vi "Begin.vi"(11 "Image Size":T1=enum."160x120") -> (0 "error out":errorcluster)   [LabVIEW 2012]
doc: "Called before other user functions, this VI is expected to open initial I/O refnums, load in file data, and do all program initialization. Notice that the <B>error out</B> terminal is simply used for data flow. Wiring it to other structures or subVIs ensures that this VI runs first."
uses:
  <vilib>/Rock Robotics/WPI/Camera/WPI_CameraImageSize.ctl
  <vilib>/Rock Robotics/WPI/DriverStation/WPI_DriverStationRobotMode2.ctl
  <vilib>/Rock Robotics/WPI/CAN/Jaguar/SubVIs/WPI_CANJaguar_BrakeCoastMode.ctl
  <vilib>/Rock Robotics/WPI/CAN/Jaguar/SubVIs/WPI_CANJaguar_SpeedReference.ctl
  <vilib>/Rock Robotics/WPI/CAN/Jaguar/SubVIs/WPI_CANJaguar_ControlMode.ctl
  <vilib>/Rock Robotics/WPI/Joystick/WPI_JoystickDeviceEnum.ctl
  <vilib>/Rock Robotics/SystemInterfaces/Typedef/FPGA_TypedefDigitalModule.ctl
  <vilib>/Rock Robotics/SystemInterfaces/DIO/FPGA_DIOChannel.ctl
  <vilib>/Rock Robotics/SystemInterfaces/DIO/FPGA_DIORelayChannel.ctl
  <vilib>/Rock Robotics/SystemInterfaces/Typedef/FPGA_TypedefSolenoidModule.ctl
  <vilib>/Rock Robotics/WPI/Solenoid/WPI_SolenoidChannel.ctl
  <vilib>/Rock Robotics/WPI/Solenoid/WPI_SolenoidValue.ctl
  Robot Global Data.vi
  <vilib>/Rock Robotics/WPI/MotorControl/WPI_MotorControlOpenCANJaguar.vi
  <vilib>/Rock Robotics/WPI/RobotDrive/WPI_RobotDriveOpen4MotorWithExistingMotors.vi
  <vilib>/Rock Robotics/WPI/Solenoid/WPI_SolenoidOpenSingle.vi
  <vilib>/Rock Robotics/WPI/Solenoid/WPI_SolenoidSetEnum.vi
  <vilib>/Rock Robotics/WPI/Compressor/WPI_CompressorGetSetRefNum.vi
  <vilib>/Rock Robotics/WPI/RobotDrive/WPI_RobotDriveOpen2MotorWithJaguar.vi
  <vilib>/Rock Robotics/SystemInterfaces/DIO/FPGA_DIOPWMChannel.ctl
  <vilib>/Rock Robotics/WPI/Camera/WPI_CameraWhite Balance Values.ctl
  <vilib>/Rock Robotics/WPI/Camera/WPI_CameraExposure Values.ctl
  <vilib>/Rock Robotics/WPI/Camera/WPI_CameraFrameRate.ctl
  <vilib>/Rock Robotics/WPI/SafetyOutput/WPI_SafetyOutputConfigMenu.ctl
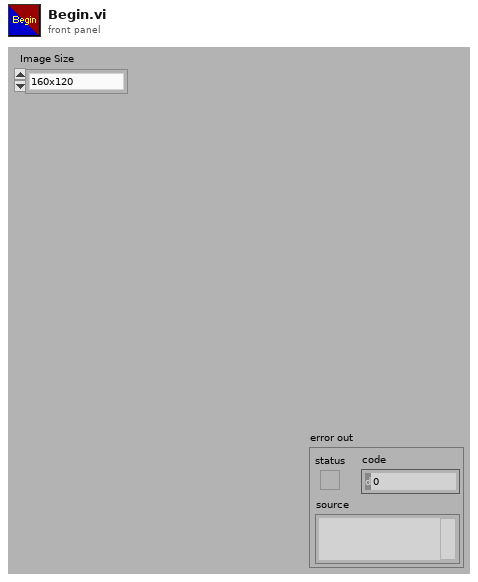
[diagram p1: front panel]
types:
  T1 = typedef "WPI_CameraImageSize.ctl" = enum16{"640x480", "320x240", "160x120"}
  T2 = typedef "WPI_SolenoidValue.ctl" = enum16{"Off", "On", "Forward", "Reverse"}
  T3 = typedef "WPI_SolenoidChannel.ctl" = enum8{"Solenoid 1", "Solenoid 2", "Solenoid 3", "Solenoid 4", "Solenoid 5", "Solenoid 6", "Solenoid 7", "Solenoid 8", "Invalid"}
  T4 = typedef "FPGA_TypedefSolenoidModule.ctl" = enum16{"Solenoid Module 1", "Solenoid Module 2"}
  T5 = typedef "FPGA_DIORelayChannel.ctl" = enum8{"Relay 1", "Relay 2", "Relay 3", "Relay 4", "Relay 5", "Relay 6", "Relay 7", "Relay 8", "Invalid"}
  T6 = typedef "FPGA_TypedefDigitalModule.ctl" = enum16{"Digital Module 1", "Digital Module 2"}
  T7 = typedef "FPGA_DIOChannel.ctl" = enum8{"DIO 1", "DIO 2", "DIO 3", "DIO 4", "DIO 5", "DIO 6", "DIO 7", "DIO 8", "DIO 9", "DIO 10", "DIO 11", "DIO 12", "DIO 13", "DIO 14", "Invalid"}
  T8 = typedef "WPI_JoystickDeviceEnum.ctl" = enum16{"USB 1", "USB 2", "USB 3", "USB 4", "Kinect 1", "Kinect 2"}
  T9 = typedef "WPI_CANJaguar_BrakeCoastMode.ctl" = enum8{"Jumper", "Brake", "Coast"}
  T10 = typedef "WPI_CANJaguar_SpeedReference.ctl" = u8
  T11 = typedef "WPI_CANJaguar_ControlMode.ctl" = enum8{"Percent VBus", "Current", "Speed", "Position", "Voltage"}
  T12 = typedef "WPI_DriverStationRobotMode2.ctl" = enum16{"Autonomous Disabled", "Autonomous Enabled", "Teleop Disabled", "Teleop Enabled", "Timeout", "Finish", "Test Disabled", "Test Enabled"}
  T13 = typedef "WPI_SafetyOutputConfigMenu.ctl" = enum16{"Enable", "Disable"}
  T14 = typedef "WPI_CameraFrameRate.ctl" = u32
  T15 = typedef "WPI_CameraExposure Values.ctl" = enum16{"Auto", "Flicker-free 50 Hz", "Flicker-free 60 Hz", "Hold current"}
  T16 = typedef "WPI_CameraWhite Balance Values.ctl" = enum16{"Auto", "Fixed indoor", "Fixed outdoor 1", "Fixed outdoor 2", "Fixed fluorescent 1", "Fixed fluorescent 2", "Hold current"}
  T17 = typedef "FPGA_DIOPWMChannel.ctl" = enum8{"PWM 1", "PWM 2", "PWM 3", "PWM 4", "PWM 5", "PWM 6", "PWM 7", "PWM 8", "PWM 9", "PWM 10", "Invalid"}
  T18 = typedef "WPI_CameraDevRef.ctl" = cluster{"Camera Address":string, "CameraStatus":errorcluster, "Acquire Image Notifier":refnum<notifier>}
  T19 = typedef "WPI_JoystickDevRef.ctl" = cluster{"Device":T8}
  T20 = typedef "WPI_RobotDriveDevRef.ctl" = cluster{"DevStatus":errorcluster, "Motors[]":T21[], "Square Inputs":bool, "Max Output":dbl, "Isochronous":bool}
  T21 = typedef "WPI_MotorControlDeviceRef.ctl" = cluster{"DeviceStatus":errorcluster, "Type":enum16{"PWM", "CAN"}, "PWM":cluster{"Digital Module":T6, "PWM Channel":T17, "DeadBand":T22}, "CAN":cluster{"Device Number":u8, "Control Mode":T11, "Semaphore":T23, "Max Vout":dbl}, "Invert":bool, "TransformRef":T24, "InvTransformRef":T24}
  T22 = typedef "WPI_PWMDeadband.ctl" = cluster{"Name":string, "maxPositivePwm":i32, "minPositivePwm":i32, "centerPwm":i32, "maxNegativePwm":i32, "minNegativePwm":i32, "angularRange":u16}
  T23 = typedef "Semaphore RefNum" = refnum<k1>
  T24 = typedef "WPI_PWMTransform_ConPane.ctl" = refnum<vi>
  T25 = typedef "WPI_SolenoidDevRef.ctl" = cluster{"DevStatus":errorcluster, "Solenoid Module":T4, "Forward Solenoid Channel":T3, "Reverse Solenoid Channel":T3}
  T26 = typedef "WPI_CompressorDevRef.ctl" = cluster{"DevStatus":errorcluster, "DigitalInputDevRef":T27, "RelayDevRef":T28}
  T27 = typedef "WPI_DigitalInputDevRef.ctl" = cluster{"DevStatus":errorcluster, "DIO Channel":T7, "Digital Module":T6}
  T28 = typedef "WPI_RelayDevRef.ctl" = cluster{"DevStatus":errorcluster, "Relay Channel":T5, "Digital Module":T6, "Relay Direction":T29}
  T29 = typedef "WPI_RelayDirection.ctl" = enum16{"Both directions", "Forward only", "Reverse only"}
  T30 = typedef "WPI_SerialPortRef.ctl" = cluster{"DevStatus":errorcluster, "Serial Port Name":refnum<visa-resource-name>}
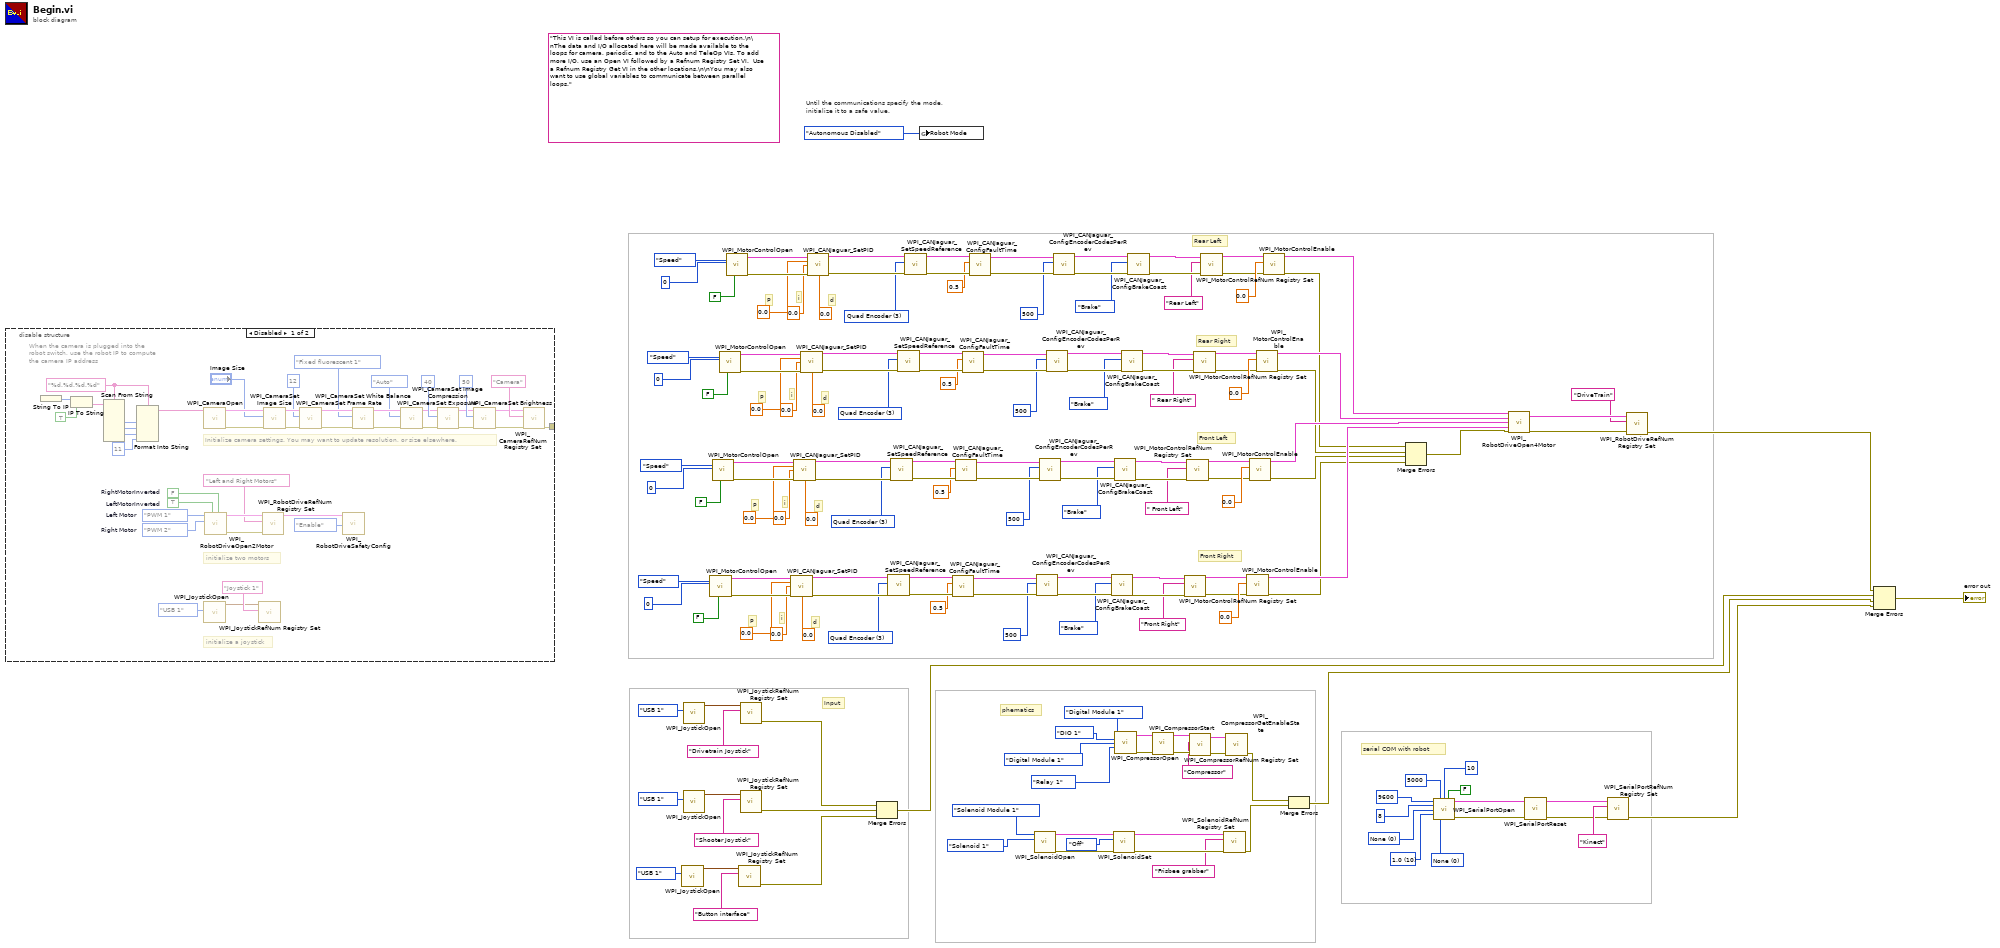
[diagram p0: block diagram]
diagram:
  w28 = u16 10 items=["1.0"=10, "1.5"=15, "2.0"=20] ("Stop Bits")
  w29 = u16 0 items=["None", "Odd", "Even", "Mark", "Space"] ("Parity")
  w32 = u16 0 items=["None", "XON/XOFF", "RTS/CTS", "XON/XOFF & RTS/CTS", "DTR/DSR", "XON/XOFF & DTR/DSR"] ("Flow Control")
  w76 = T10 3 items=["Encoder"=0, "Inv Encoder"=2, "Quad Encoder"=3, "None"=255] ("Speed Reference")
  w102 = T10 3 items=["Encoder"=0, "Inv Encoder"=2, "Quad Encoder"=3, "None"=255] ("Speed Reference")
  w128 = T10 3 items=["Encoder"=0, "Inv Encoder"=2, "Quad Encoder"=3, "None"=255] ("Speed Reference")
  w154 = T10 3 items=["Encoder"=0, "Inv Encoder"=2, "Quad Encoder"=3, "None"=255] ("Speed Reference")
  (unwired) "This VI is called before others so you can setup for execution.\n\nThe data and I/O allocated here will be made available to the loops for camera, periodic, and to the Auto and TeleOp VIs. To add more I/O, use an Open VI followed by a Refnum Registry Set VI.  Use a Refnum Registry Get VI in the other locations.\n\nYou may also want to use global variables to communicate between parallel loops."
  # "phematics"
  # "serial COM with robot"
  # "Input"
  # "Front Right"
  # "Front Left"
  # "Rear Right"
  # "Rear Left"
  # "d"
  # "i"
  # "P"
  # "d"
  # "i"
  # "P"
  # "d"
  # "i"
  # "P"
  # "d"
  # "i"
  # "P"
  # "Until the communications specify the mode,\ninitialize it to a safe value."
  n1 = disable-structure shown="Disabled" {
    disable-tunnel: [w169 _] -> _
    frame Disabled {
      w176 = "%d.%d.%d.%d" ("format string")
      w187 = FPGA_DIOPWMChannel."PWM 2"  # Right Motor
      w188 = FPGA_DIOPWMChannel."PWM 1"  # Left Motor
      w210 = TRUE  # LeftMotorInverted
      w211 = FALSE  # RightMotorInverted
      # "initialize a joystick"
      # "When the camera is plugged into the\nrobot switch, use the robot IP to compute\nthe camera IP address"
      # "initialize two motors"
      # "Initialize camera settings. You may want to update resolution, or size elsewhere."
      n2 = String To IP() -> (0:w183:u32)  [unwired: 1 in]
      n3 = IP To String(1:TRUE ("dot notation? (F)"), 2:w183) -> (0:w181:string)
      n4 = Scan From String(format string=w176, input string=w181) -> (output 1=w180:i32, output 2=w179:i32, output 3=w178:i32)  [unwired: 7 in, 3 out]
      n5 = Format Into String(format string=w176, w180, w179, w178, 11 ("Compression")) -> (resulting string=w173:string)  [unwired: 2 in, 1 out]
      n6 = call <vilib>:"WPI_CameraOpen.vi"("Camera Address"=w173) -> ("error out"=w197:errorcluster, "CameraDevRef"=w198:T18)  [unwired: 1 in, 8 out]
      n7 = call <vilib>:"WPI_JoystickOpen.vi"("JoystickDevice"=WPI_JoystickDeviceEnum."USB 1") -> ("JoystickDevRef"=w171:T19)  [unwired: 10 in]
      n8 = call-poly <vilib>:"WPI_RobotDriveOpen2Motor.vi"("Right Motor Inverted"=w211, "Left Motor Inverted"=w210, "Right Motor"=w187, "Left Motor"=w188) -> ("error out"=w206:errorcluster, "RobotDriveDevRef"=w208:T20)  [unwired: 1 in, 5 out]
      n9 = call <vilib>:"WPI_JoystickRefNum Registry Set.vi"("refnum name"="Joystick 1", "JoystickDevRef"=w171) -> ()  [unwired: 8 in, 2 out]
      n10 = call <vilib>:"WPI_RobotDriveRefNum Registry Set.vi"("error in (no error)"=w206, "refnum name"="Left and Right Motors", "RobotDriveDevRef"=w208) -> ("RobotDriveDevRef"=w175:T20)  [unwired: 8 out]
      n11 = call <vilib>:"WPI_CameraSet Image Size.vi"("error in (no error)"=w197, "Image Size"="Image Size", "CameraDevRef"=w198) -> ("error out"=w196:errorcluster, "CameraDevRef Out"=w199:T18)  [unwired: 7 out]
      n12 = call <vilib>:"WPI_CameraSet Frame Rate.vi"("error in (no error)"=w196, "Frame Rate (fps)"=T14 12, "CameraDevRef"=w199) -> ("error out"=w195:errorcluster, "CameraDevRef Out"=w201:T18)  [unwired: 7 out]
      n13 = call <vilib>:"WPI_RobotDriveSafetyConfig.vi"("mode"=WPI_SafetyOutputConfigMenu."Enable", "RobotDriveDevRef"=w175) -> ()  [unwired: 8 in, 2 out]
      n14 = call <vilib>:"WPI_CameraSet White Balance.vi"("error in (no error)"=w195, "White Balance"=WPI_CameraWhite_Balance_Values."Fixed fluorescent 1", "CameraDevRef"=w201) -> ("error out"=w194:errorcluster, "CameraDevRef Out"=w200:T18)  [unwired: 7 out]
      n15 = call <vilib>:"WPI_CameraSet Exposure.vi"("error in (no error)"=w194, "Exposure"=WPI_CameraExposure_Values."Auto", "CameraDevRef"=w200) -> ("error out"=w193:errorcluster, "CameraDevRef Out"=w203:T18)  [unwired: 7 out]
      n16 = call <vilib>:"WPI_CameraSet Image Compression.vi"("error in (no error)"=w193, "Compression"=40, "CameraDevRef"=w203) -> ("error out"=w192:errorcluster, "CameraDevRef Out"=w202:T18)  [unwired: 7 out]
      n17 = call <vilib>:"WPI_CameraSet Brightness.vi"("error in (no error)"=w192, "Brightness"=50, "CameraDevRef"=w202) -> ("error out"=w190:errorcluster, "CameraDevRef Out"=w191:T18)  [unwired: 7 out]
      n18 = call <vilib>:"WPI_CameraRefNum Registry Set.vi"("error in (no error)"=w190, "refnum name"="Camera", "CameraDevRef"=w191) -> ("error out"=w169:errorcluster)  [unwired: 8 out]
    }
    frame Enabled {
    }
  }
  n19 = call <vilib>:"WPI_JoystickOpen.vi"("JoystickDevice"=WPI_JoystickDeviceEnum."USB 1") -> ("JoystickDevRef"=w45:T19)  [unwired: 10 in]
  n20 = call <vilib>:"WPI_JoystickOpen.vi"("JoystickDevice"=WPI_JoystickDeviceEnum."USB 1") -> ("JoystickDevRef"=w51:T19)  [unwired: 10 in]
  n21 = call <vilib>:"WPI_JoystickOpen.vi"("JoystickDevice"=WPI_JoystickDeviceEnum."USB 1") -> ("JoystickDevRef"=w48:T19)  [unwired: 10 in]
  n22 = call-poly <vilib>:"WPI_MotorControlOpen.vi"("Invert"=FALSE, "Device Number"=u8 0, "Control Mode"=WPI_CANJaguar_ControlMode."Speed") -> ("error out"=w83:errorcluster, "MotorControlDeviceRef"=w82:T21)  [unwired: 7 in]
  n23 = call-poly <vilib>:"WPI_MotorControlOpen.vi"("Invert"=FALSE, "Device Number"=u8 0, "Control Mode"=WPI_CANJaguar_ControlMode."Speed") -> ("error out"=w109:errorcluster, "MotorControlDeviceRef"=w108:T21)  [unwired: 7 in]
  n24 = call-poly <vilib>:"WPI_MotorControlOpen.vi"("Invert"=FALSE, "Device Number"=u8 0, "Control Mode"=WPI_CANJaguar_ControlMode."Speed") -> ("error out"=w135:errorcluster, "MotorControlDeviceRef"=w134:T21)  [unwired: 7 in]
  n25 = call-poly <vilib>:"WPI_MotorControlOpen.vi"("Invert"=FALSE, "Device Number"=u8 0, "Control Mode"=WPI_CANJaguar_ControlMode."Speed") -> ("error out"=w161:errorcluster, "MotorControlDeviceRef"=w160:T21)  [unwired: 7 in]
  n26 = call <vilib>:"WPI_JoystickRefNum Registry Set.vi"("refnum name"="Button interface", "JoystickDevRef"=w45) -> ("error out"=w40:errorcluster)  [unwired: 8 in, 1 out]
  n27 = call <vilib>:"WPI_JoystickRefNum Registry Set.vi"("refnum name"="Drivetrain Joystick", "JoystickDevRef"=w51) -> ("error out"=w42:errorcluster)  [unwired: 8 in, 1 out]
  n28 = call <vilib>:"WPI_JoystickRefNum Registry Set.vi"("refnum name"="Shooter Joystick", "JoystickDevRef"=w48) -> ("error out"=w41:errorcluster)  [unwired: 8 in, 1 out]
  n29 = call <vilib>:"WPI_CANJaguar_SetPID.vi"("CAN Jaguar Ref"=w82, "P"=0.0, "I"=0.0, "D"=0.0, "error in (no error)"=w83) -> ("CAN Jaguar Ref Out"=w89:T21, "error out"=w88:errorcluster)  [unwired: 9 in]
  n30 = call <vilib>:"WPI_CANJaguar_SetPID.vi"("CAN Jaguar Ref"=w108, "P"=0.0, "I"=0.0, "D"=0.0, "error in (no error)"=w109) -> ("CAN Jaguar Ref Out"=w115:T21, "error out"=w114:errorcluster)  [unwired: 9 in]
  n31 = call <vilib>:"WPI_CANJaguar_SetPID.vi"("CAN Jaguar Ref"=w134, "P"=0.0, "I"=0.0, "D"=0.0, "error in (no error)"=w135) -> ("CAN Jaguar Ref Out"=w141:T21, "error out"=w140:errorcluster)  [unwired: 9 in]
  n32 = call <vilib>:"WPI_CANJaguar_SetPID.vi"("CAN Jaguar Ref"=w160, "P"=0.0, "I"=0.0, "D"=0.0, "error in (no error)"=w161) -> ("CAN Jaguar Ref Out"=w167:T21, "error out"=w166:errorcluster)  [unwired: 9 in]
  n33 = Merge Errors(w42, w41, w40) -> (w3:errorcluster)
  n34 = call <vilib>:"WPI_CANJaguar_SetSpeedReference.vi"("error in (no error)"=w88, "Speed Reference"=w76, "CAN Jaguar Ref"=w89) -> ("error out"=w87:errorcluster, "CAN Jaguar Ref Out"=w86:T21)  [unwired: 7 in]
  n35 = call <vilib>:"WPI_CANJaguar_SetSpeedReference.vi"("error in (no error)"=w114, "Speed Reference"=w102, "CAN Jaguar Ref"=w115) -> ("error out"=w113:errorcluster, "CAN Jaguar Ref Out"=w112:T21)  [unwired: 7 in]
  n36 = call <vilib>:"WPI_CANJaguar_SetSpeedReference.vi"("error in (no error)"=w140, "Speed Reference"=w128, "CAN Jaguar Ref"=w141) -> ("error out"=w139:errorcluster, "CAN Jaguar Ref Out"=w138:T21)  [unwired: 7 in]
  n37 = call <vilib>:"WPI_CANJaguar_SetSpeedReference.vi"("error in (no error)"=w166, "Speed Reference"=w154, "CAN Jaguar Ref"=w167) -> ("error out"=w165:errorcluster, "CAN Jaguar Ref Out"=w164:T21)  [unwired: 7 in]
  n38 = global write "Robot Global Data.vi" "Robot Mode"(WPI_DriverStationRobotMode2."Autonomous Disabled" ("Robot Mode")) -> ()
  n39 = call <vilib>:"WPI_CANJaguar_ConfigFaultTime.vi"("error in (no error)"=w87, "Fault Time (s)"=0.5, "CAN Jaguar Ref"=w86) -> ("error out"=w84:errorcluster, "CAN Jaguar Ref Out"=w85:T21)  [unwired: 7 in]
  n40 = call <vilib>:"WPI_CANJaguar_ConfigFaultTime.vi"("error in (no error)"=w113, "Fault Time (s)"=0.5, "CAN Jaguar Ref"=w112) -> ("error out"=w110:errorcluster, "CAN Jaguar Ref Out"=w111:T21)  [unwired: 7 in]
  n41 = call <vilib>:"WPI_CANJaguar_ConfigFaultTime.vi"("error in (no error)"=w139, "Fault Time (s)"=0.5, "CAN Jaguar Ref"=w138) -> ("error out"=w136:errorcluster, "CAN Jaguar Ref Out"=w137:T21)  [unwired: 7 in]
  n42 = call <vilib>:"WPI_CANJaguar_ConfigFaultTime.vi"("error in (no error)"=w165, "Fault Time (s)"=0.5, "CAN Jaguar Ref"=w164) -> ("error out"=w162:errorcluster, "CAN Jaguar Ref Out"=w163:T21)  [unwired: 7 in]
  n43 = call-poly <vilib>:"WPI_SolenoidOpen.vi"("Solenoid Channel"=WPI_SolenoidChannel."Solenoid 1", "Solenoid Module (Module 1)"=FPGA_TypedefSolenoidModule."Solenoid Module 1") -> ("error out"=w11:errorcluster, "SolenoidDevRef"=w13:T25)  [unwired: 8 in]
  n44 = call <vilib>:"WPI_CANJaguar_ConfigEncoderCodesPerRev.vi"("error in (no error)"=w84, "Encoder Codes Per Rev"=u16 500, "CAN Jaguar Ref"=w85) -> ("error out"=w73:errorcluster, "CAN Jaguar Ref Out"=w72:T21)  [unwired: 7 in]
  n45 = call <vilib>:"WPI_CANJaguar_ConfigEncoderCodesPerRev.vi"("error in (no error)"=w110, "Encoder Codes Per Rev"=u16 500, "CAN Jaguar Ref"=w111) -> ("error out"=w99:errorcluster, "CAN Jaguar Ref Out"=w98:T21)  [unwired: 7 in]
  n46 = call <vilib>:"WPI_CANJaguar_ConfigEncoderCodesPerRev.vi"("error in (no error)"=w136, "Encoder Codes Per Rev"=u16 500, "CAN Jaguar Ref"=w137) -> ("error out"=w125:errorcluster, "CAN Jaguar Ref Out"=w124:T21)  [unwired: 7 in]
  n47 = call <vilib>:"WPI_CANJaguar_ConfigEncoderCodesPerRev.vi"("error in (no error)"=w162, "Encoder Codes Per Rev"=u16 500, "CAN Jaguar Ref"=w163) -> ("error out"=w151:errorcluster, "CAN Jaguar Ref Out"=w150:T21)  [unwired: 7 in]
  n48 = call <vilib>:"WPI_CANJaguar_ConfigBrakeCoast.vi"("error in (no error)"=w73, "Brake / Coast Mode"=WPI_CANJaguar_BrakeCoastMode."Brake", "CAN Jaguar Ref"=w72) -> ("error out"=w69:errorcluster, "CAN Jaguar Ref Out"=w70:T21)  [unwired: 7 in]
  n49 = call-poly <vilib>:"WPI_SolenoidSet.vi"("error in (no error)"=w11, "Value"=WPI_SolenoidValue."Off", "SolenoidDevRef"=w13) -> ("error out"=w10:errorcluster, "SolenoidDevRef"=w9:T25)  [unwired: 7 in]
  n50 = call <vilib>:"WPI_CANJaguar_ConfigBrakeCoast.vi"("error in (no error)"=w99, "Brake / Coast Mode"=WPI_CANJaguar_BrakeCoastMode."Brake", "CAN Jaguar Ref"=w98) -> ("error out"=w95:errorcluster, "CAN Jaguar Ref Out"=w96:T21)  [unwired: 7 in]
  n51 = call <vilib>:"WPI_CompressorOpen.vi"("Pressure Switch Digital Module (Module 1)"=FPGA_TypedefDigitalModule."Digital Module 1", "Pressure Switch DIO Channel"=FPGA_DIOChannel."DIO 1", "Relay Digital Module (Module 1)"=FPGA_TypedefDigitalModule."Digital Module 1", "Relay Channel"=FPGA_DIORelayChannel."Relay 1") -> ("CompressorDevRef"=w22:T26, "error out"=w21:errorcluster)  [unwired: 10 in]
  n52 = call <vilib>:"WPI_CANJaguar_ConfigBrakeCoast.vi"("error in (no error)"=w125, "Brake / Coast Mode"=WPI_CANJaguar_BrakeCoastMode."Brake", "CAN Jaguar Ref"=w124) -> ("error out"=w121:errorcluster, "CAN Jaguar Ref Out"=w122:T21)  [unwired: 7 in]
  n53 = call <vilib>:"WPI_CANJaguar_ConfigBrakeCoast.vi"("error in (no error)"=w151, "Brake / Coast Mode"=WPI_CANJaguar_BrakeCoastMode."Brake", "CAN Jaguar Ref"=w150) -> ("error out"=w147:errorcluster, "CAN Jaguar Ref Out"=w148:T21)  [unwired: 7 in]
  n54 = call <vilib>:"WPI_CompressorStart.vi"("error in (no error)"=w21, "CompressorDevRef"=w22) -> ("error out"=w26:errorcluster, "CompressorDevRef"=w25:T26)  [unwired: 8 in]
  n55 = call <vilib>:"WPI_MotorControlRefNum Registry Set.vi"("error in (no error)"=w69, "refnum name"="Front Right", "MotorControlDevRef"=w70) -> ("error out"=w64:errorcluster, "MotorControlDevRef"=w66:T21)  [unwired: 7 in]
  n56 = call <vilib>:"WPI_MotorControlRefNum Registry Set.vi"("error in (no error)"=w95, "refnum name"=" Front Left", "MotorControlDevRef"=w96) -> ("error out"=w90:errorcluster, "MotorControlDevRef"=w92:T21)  [unwired: 7 in]
  n57 = call <vilib>:"WPI_CompressorRefNum Registry Set.vi"("error in (no error)"=w26, "refnum name"="Compressor", "CompressorDevRef"=w25) -> ("error out"=w24:errorcluster, "CompressorDevRef"=w23:T26)  [unwired: 7 in]
  n58 = call <vilib>:"WPI_MotorControlRefNum Registry Set.vi"("error in (no error)"=w121, "refnum name"=" Rear Right", "MotorControlDevRef"=w122) -> ("error out"=w116:errorcluster, "MotorControlDevRef"=w118:T21)  [unwired: 7 in]
  n59 = call <vilib>:"WPI_MotorControlRefNum Registry Set.vi"("error in (no error)"=w147, "refnum name"="Rear Left", "MotorControlDevRef"=w148) -> ("error out"=w142:errorcluster, "MotorControlDevRef"=w144:T21)  [unwired: 7 in]
  n60 = call <vilib>:"WPI_SolenoidRefNum Registry Set.vi"("error in (no error)"=w10, "refnum name"="Frisbee grabber", "SolenoidDevRef"=w9) -> ("error out"=w6:errorcluster)  [unwired: 7 in, 1 out]
  n61 = call <vilib>:"WPI_CompressorGetEnableState.vi"("error in (no error)"=w24, "CompressorDevRef"=w23) -> ("error out"=w7:errorcluster)  [unwired: 6 in, 3 out]
  n62 = call <vilib>:"WPI_MotorControlEnable.vi"("error in (no error)"=w64, "Encoder Initial Position"=0.0, "CAN Jaguar Ref"=w66) -> ("error out"=w57:errorcluster, "CAN Jaguar Ref Out"=w60:T21)  [unwired: 7 in]
  n63 = call <vilib>:"WPI_MotorControlEnable.vi"("error in (no error)"=w90, "Encoder Initial Position"=0.0, "CAN Jaguar Ref"=w92) -> ("error out"=w56:errorcluster, "CAN Jaguar Ref Out"=w61:T21)  [unwired: 7 in]
  n64 = call <vilib>:"WPI_MotorControlEnable.vi"("error in (no error)"=w116, "Encoder Initial Position"=0.0, "CAN Jaguar Ref"=w118) -> ("error out"=w58:errorcluster, "CAN Jaguar Ref Out"=w62:T21)  [unwired: 7 in]
  n65 = call <vilib>:"WPI_MotorControlEnable.vi"("error in (no error)"=w142, "Encoder Initial Position"=0.0, "CAN Jaguar Ref"=w144) -> ("error out"=w59:errorcluster, "CAN Jaguar Ref Out"=w63:T21)  [unwired: 7 in]
  n66 = Merge Errors(w7, w6) -> (w2:errorcluster)
  n67 = Merge Errors(w59, w58, w56, w57) -> (w55:errorcluster)
  n68 = call <vilib>:"WPI_SerialPortOpen.vi"("Baud Rate"=u32 9600, "Timeout Value (ms)"=u32 5000, "Termination Char (0xA = '\\n' = LF)"=u8 10 ("Termination Char (0xA = '\\n' = LF)"), "Enable Termination Char? (T)"=FALSE, "Data Bits"=u16 8, "Parity"=w29, "Stop Bits"=w28, "Flow Control"=w32) -> ("SerialPortRef"=w39:T30, "error out"=w38:errorcluster)  [unwired: 6 in]
  n69 = call-poly <vilib>:"WPI_RobotDriveOpen4Motor.vi"("Rear Left Motor Dev Ref"=w63, "Rear Right Motor Dev Ref"=w62, "Front Left Motor Dev Ref"=w61, "Front Right Motor Dev Ref"=w60, "error in (no error)"=w55) -> ("RobotDriveDevRef"=w54:T20, "error out"=w53:errorcluster)  [unwired: 9 in]
  n70 = call <vilib>:"WPI_SerialPortReset.vi"("error in (no error)"=w38, "SerialPortRef"=w39) -> ("error out"=w34:errorcluster, "SerialPortRef"=w33:T30)  [unwired: 8 in]
  n71 = call <vilib>:"WPI_SerialPortRefNum Registry Set.vi"("error in (no error)"=w34, "refnum name"="Kinect", "SerialPortRef"=w33) -> ("error out"=w1:errorcluster)  [unwired: 7 in, 1 out]
  n72 = call <vilib>:"WPI_RobotDriveRefNum Registry Set.vi"("error in (no error)"=w53, "refnum name"="DriveTrain", "RobotDriveDevRef"=w54) -> ("error out"=w4:errorcluster)  [unwired: 7 in, 1 out]
  n73 = Merge Errors(w4, w3, w2, w1) -> (→"error out":errorcluster)
